vi "HFRR ADV v08.vi"() -> ()   [LabVIEW 2025] (continued)
            n1801 = String To Path(string=w2038) -> (path=w2046:path)
            n1802 = case shown="True" w2037 {
              tunnel: [w2053 w2054] -> w2041
              frame False {
                n1803 = local read "string1"() -> (w2053:string)
              }
              frame True {
                n1804 = local read "String Indicator 4"() -> (w2054:string)
              }
            }
            n1805 = Open/Create/Replace File "Open File"(file path (use dialog)=w2048) -> (refnum out=w2044:refnum<file>)  [unwired: 5 in, 2 out]
            n1806 = Open/Create/Replace File "Open File"(file path (use dialog)=w2047) -> (refnum out=w2043:refnum<file>)  [unwired: 5 in, 2 out]
            n1807 = Open/Create/Replace File "Open File"(file path (use dialog)=w2046) -> (refnum out=w2042:refnum<file>)  [unwired: 5 in, 2 out]
            n1808 = while {
              tunnel: w2044 -> [w2066]
              i -> [w2062]
              stop <- w2061 continue-if-true
              (unwired) TRUE ("line mode (F)")
              n1809 = Read from Text File "Read File"(file (use dialog)=w2066) -> (text=w2063:string)  [unwired: 3 in, 3 out]
              n1810 = local write "Numeric 11"(w2062) -> ()
              n1811 = String Length(string=w2063) -> (length=w2065:i32)
              n1812 = Greater?(x=w2065, y=1) -> (0:w2061:bool)
            }
            n1813 = while {
              tunnel: w2043 -> [w2072]
              i -> [w2068]
              stop <- w2067 continue-if-true
              (unwired) TRUE ("line mode (F)")
              n1814 = Read from Text File "Read File"(file (use dialog)=w2072) -> (text=w2069:string)  [unwired: 3 in, 3 out]
              n1815 = local write "Numeric 12"(w2068) -> ()
              n1816 = String Length(string=w2069) -> (length=w2071:i32)
              n1817 = Greater?(x=w2071, y=1) -> (0:w2067:bool)
            }
            n1818 = while {
              tunnel: w2042 -> [w2078]
              i -> [w2074]
              stop <- w2073 continue-if-true
              (unwired) TRUE ("line mode (F)")
              n1819 = Read from Text File "Read File"(file (use dialog)=w2078) -> (text=w2075:string)  [unwired: 3 in, 3 out]
              n1820 = local write "Numeric 13"(w2074) -> ()
              n1821 = String Length(string=w2075) -> (length=w2077:i32)
              n1822 = Greater?(x=w2077, y=1) -> (0:w2073:bool)
            }
            n1823 = String To Path(string=w2041) -> (path=w2049:path)
            n1824 = Open/Create/Replace File "Open File"(file path (use dialog)=w2049) -> (refnum out=w2045:refnum<file>)  [unwired: 5 in, 2 out]
            n1825 = while {
              tunnel: w2045 -> [w2060]
              i -> [w2056]
              stop <- w2055 continue-if-true
              (unwired) TRUE ("line mode (F)")
              n1826 = Read from Text File "Read File"(file (use dialog)=w2060) -> (text=w2057:string)  [unwired: 3 in, 3 out]
              n1827 = local write "Numeric 8"(w2056) -> ()
              n1828 = String Length(string=w2057) -> (length=w2059:i32)
              n1829 = Greater?(x=w2059, y=1) -> (0:w2055:bool)
            }
          }
          frame #1 {
            w2230 = FALSE ("ACTUAL   MERGE")
            # "Sample Temp"
            # "ECR"
            # "COF"
            # "Time\nCOF\nFF\nTemp"
            n1830 = case shown="True" w2103 {
              tunnel: [w2250 w2251] -> w2104
              frame False {
                n1831 = local read "string1"() -> (w2250:string)
              }
              frame True {
                n1832 = local read "String Indicator 4"() -> (w2251:string)
              }
            }
            n1833 = local read "string1 3"() -> (w2148:string)
            n1834 = String To Path(string=w2104) -> (path=w2235:path)
            n1835 = String To Path(string=w2148) -> (path=w2246:path)
            n1836 = local read "Numeric 12"() -> (w2232:i32)
            n1837 = local read "Numeric 8"() -> (w2234:i32)
            n1838 = local read "string1 2"() -> (w2149:string)
            n1839 = local read "string1 4"() -> (w2147:string)
            n1840 = Open/Create/Replace File "Open File"(file path (use dialog)=w2235) -> (refnum out=w2249:refnum<file>, error out=w2248:errorcluster)  [unwired: 5 in, 1 out]
            n1841 = Open/Create/Replace File "Open File"(file path (use dialog)=w2246) -> (refnum out=w2242:refnum<file>, error out=w2243:errorcluster)  [unwired: 5 in, 1 out]
            n1842 = for {
              N: w2234 -> [_]
              tunnel: w2249 -> [w2397]
              tunnel: w2248 -> [w2396]
              tunnel: [w2386] -> w2161 mode=indexing
              tunnel: [w2384] -> w2218 mode=indexing
              tunnel: [w2385] -> w2213 mode=indexing
              tunnel: w2230 -> [_]
              tunnel: [w2378] -> w2215 mode=indexing
              tunnel: [w2374] -> w2184 mode=indexing
              tunnel: [w2370] -> w2159 mode=indexing
              tunnel: [w2366] -> w2140 mode=indexing
              tunnel: [w2361] -> w2100 mode=indexing
              (unwired) TRUE ("line mode (F)")
              # "freq"
              # "Stroke"
              # "Time"
              # "CoF"
              # "Humidity"
              # "Temp"
              # "Air Temp"
              # "ECR"
              n1843 = Read from Text File "Read File"(file (use dialog)=w2397, error in=w2396) -> (text=w2362:string)  [unwired: 2 in, 3 out]
              n1844 = local write "String 6"(w2362) -> ()
              n1845 = String Subset(string=w2362, offset (0)=0, length (rest)=14 ("length (rest)")) -> (substring=w2390:string)
              n1846 = String Subset(string=w2362, offset (0)=35, length (rest)=9 ("length (rest)")) -> (substring=w2387:string)
              n1847 = String Subset(string=w2362, offset (0)=15, length (rest)=9 ("length (rest)")) -> (substring=w2393:string)
              n1848 = Fract/Exp String To Number(string=w2390) -> (number=w2386:dbl)  [unwired: 3 in, 1 out]
              n1849 = Fract/Exp String To Number(string=w2387) -> (number=w2385:dbl)  [unwired: 3 in, 1 out]
              n1850 = Fract/Exp String To Number(string=w2393) -> (number=w2384:dbl)  [unwired: 3 in, 1 out]
              n1851 = String Subset(string=w2362, offset (0)=85, length (rest)=9 ("length (rest)")) -> (substring=w2363:string)
              n1852 = String Subset(string=w2362, offset (0)=25, length (rest)=9 ("length (rest)")) -> (substring=w2369:string)
              n1853 = String Subset(string=w2362, offset (0)=55, length (rest)=9 ("length (rest)")) -> (substring=w2371:string)
              n1854 = String Subset(string=w2362, offset (0)=45, length (rest)=9 ("length (rest)")) -> (substring=w2377:string)
              n1855 = String Subset(string=w2362, offset (0)=65, length (rest)=9 ("length (rest)")) -> (substring=w2383:string)
              n1856 = Fract/Exp String To Number(string=w2369) -> (number=w2366:dbl)  [unwired: 3 in, 1 out]
              n1857 = Fract/Exp String To Number(string=w2363) -> (number=w2361:dbl)  [unwired: 3 in, 1 out]
              n1858 = Fract/Exp String To Number(string=w2371) -> (number=w2370:dbl)  [unwired: 3 in, 1 out]
              n1859 = Fract/Exp String To Number(string=w2377) -> (number=w2374:dbl)  [unwired: 3 in, 1 out]
              n1860 = Fract/Exp String To Number(string=w2383) -> (number=w2380:dbl)  [unwired: 3 in, 1 out]
              n1861 = Add(x=w2380, y=0.0) -> (x+y=w2378:dbl)
            }
            n1862 = for {
              N: w2232 -> [_]
              tunnel: w2243 -> [w2323]
              tunnel: w2242 -> [w2322]
              tunnel: [w2312] -> w2201 mode=indexing
              tunnel: [w2310] -> w2199 mode=indexing
              tunnel: [w2311] -> w2195 mode=indexing
              tunnel: w2230 -> [_]
              tunnel: [w2304] -> w2197 mode=indexing
              tunnel: [w2300] -> w2179 mode=indexing
              tunnel: [w2296] -> w2155 mode=indexing
              tunnel: [w2293] -> w2136 mode=indexing
              tunnel: [w2289] -> w2095 mode=indexing
              (unwired) 9 ("length (rest)")
              (unwired) 9 ("length (rest)")
              (unwired) TRUE ("line mode (F)")
              n1863 = Read from Text File "Read File"(file (use dialog)=w2322, error in=w2323) -> (text=w2290:string)  [unwired: 2 in, 3 out]
              n1864 = local write "String 8"(w2290) -> ()
              n1865 = String Subset(string=w2290, offset (0)=85) -> (substring=w2292:string)  [unwired: 1 in]
              n1866 = String Subset(string=w2290, offset (0)=35, length (rest)=9 ("length (rest)")) -> (substring=w2313:string)
              n1867 = String Subset(string=w2290, offset (0)=55, length (rest)=9 ("length (rest)")) -> (substring=w2298:string)
              n1868 = String Subset(string=w2290, offset (0)=25) -> (substring=w2294:string)  [unwired: 1 in]
              n1869 = String Subset(string=w2290, offset (0)=15, length (rest)=9 ("length (rest)")) -> (substring=w2319:string)
              n1870 = String Subset(string=w2290, offset (0)=0, length (rest)=14 ("length (rest)")) -> (substring=w2316:string)
              n1871 = String Subset(string=w2290, offset (0)=45, length (rest)=9 ("length (rest)")) -> (substring=w2303:string)
              n1872 = String Subset(string=w2290, offset (0)=65, length (rest)=9 ("length (rest)")) -> (substring=w2309:string)
              n1873 = Fract/Exp String To Number(string=w2292) -> (number=w2289:dbl)  [unwired: 3 in, 1 out]
              n1874 = Fract/Exp String To Number(string=w2313) -> (number=w2311:dbl)  [unwired: 3 in, 1 out]
              n1875 = Fract/Exp String To Number(string=w2298) -> (number=w2296:dbl)  [unwired: 3 in, 1 out]
              n1876 = Fract/Exp String To Number(string=w2294) -> (number=w2293:dbl)  [unwired: 3 in, 1 out]
              n1877 = Fract/Exp String To Number(string=w2319) -> (number=w2310:dbl)  [unwired: 3 in, 1 out]
              n1878 = Fract/Exp String To Number(string=w2316) -> (number=w2312:dbl)  [unwired: 3 in, 1 out]
              n1879 = Fract/Exp String To Number(string=w2303) -> (number=w2300:dbl)  [unwired: 3 in, 1 out]
              n1880 = Fract/Exp String To Number(string=w2309) -> (number=w2306:dbl)  [unwired: 3 in, 1 out]
              n1881 = Add(x=w2306, y=0.0) -> (x+y=w2304:dbl)
            }
            n1882 = String To Path(string=w2149) -> (path=w2247:path)
            n1883 = String To Path(string=w2147) -> (path=w2241:path)
            n1884 = local read "Numeric 11"() -> (w2231:i32)
            n1885 = local read "Numeric 13"() -> (w2233:i32)
            n1886 = Open/Create/Replace File "Open File"(file path (use dialog)=w2247) -> (refnum out=w2245:refnum<file>, error out=w2244:errorcluster)  [unwired: 5 in, 1 out]
            n1887 = Open/Create/Replace File "Open File"(file path (use dialog)=w2241) -> (refnum out=w2240:refnum<file>, error out=w2239:errorcluster)  [unwired: 5 in, 1 out]
            n1888 = for {
              N: w2231 -> [_]
              tunnel: w2245 -> [w2360]
              tunnel: w2244 -> [w2359]
              tunnel: [w2349] -> w2211 mode=indexing
              tunnel: [w2347] -> w2209 mode=indexing
              tunnel: [w2348] -> w2204 mode=indexing
              tunnel: w2230 -> [_]
              tunnel: [w2341] -> w2206 mode=indexing
              tunnel: [w2337] -> w2182 mode=indexing
              tunnel: [w2333] -> w2157 mode=indexing
              tunnel: [w2329] -> w2138 mode=indexing
              tunnel: [w2324] -> w2096 mode=indexing
              (unwired) TRUE ("line mode (F)")
              n1889 = Read from Text File "Read File"(file (use dialog)=w2360, error in=w2359) -> (text=w2325:string)  [unwired: 2 in, 3 out]
              n1890 = local write "String 7"(w2325) -> ()
              n1891 = String Subset(string=w2325, offset (0)=85, length (rest)=9 ("length (rest)")) -> (substring=w2328:string)
              n1892 = String Subset(string=w2325, offset (0)=35, length (rest)=9 ("length (rest)")) -> (substring=w2350:string)
              n1893 = String Subset(string=w2325, offset (0)=55, length (rest)=9 ("length (rest)")) -> (substring=w2336:string)
              n1894 = String Subset(string=w2325, offset (0)=25, length (rest)=9 ("length (rest)")) -> (substring=w2330:string)
              n1895 = String Subset(string=w2325, offset (0)=45, length (rest)=9 ("length (rest)")) -> (substring=w2338:string)
              n1896 = String Subset(string=w2325, offset (0)=0, length (rest)=14 ("length (rest)")) -> (substring=w2353:string)
              n1897 = String Subset(string=w2325, offset (0)=15, length (rest)=9 ("length (rest)")) -> (substring=w2356:string)
              n1898 = String Subset(string=w2325, offset (0)=65, length (rest)=9 ("length (rest)")) -> (substring=w2342:string)
              n1899 = Fract/Exp String To Number(string=w2328) -> (number=w2324:dbl)  [unwired: 3 in, 1 out]
              n1900 = Fract/Exp String To Number(string=w2350) -> (number=w2348:dbl)  [unwired: 3 in, 1 out]
              n1901 = Fract/Exp String To Number(string=w2336) -> (number=w2333:dbl)  [unwired: 3 in, 1 out]
              n1902 = Fract/Exp String To Number(string=w2330) -> (number=w2329:dbl)  [unwired: 3 in, 1 out]
              n1903 = Fract/Exp String To Number(string=w2338) -> (number=w2337:dbl)  [unwired: 3 in, 1 out]
              n1904 = Fract/Exp String To Number(string=w2353) -> (number=w2349:dbl)  [unwired: 3 in, 1 out]
              n1905 = Fract/Exp String To Number(string=w2356) -> (number=w2347:dbl)  [unwired: 3 in, 1 out]
              n1906 = Fract/Exp String To Number(string=w2342) -> (number=w2345:dbl)  [unwired: 3 in, 1 out]
              n1907 = Add(x=w2345, y=0.0) -> (x+y=w2341:dbl)
            }
            n1908 = for {
              N: w2233 -> [_]
              tunnel: w2240 -> [w2288]
              tunnel: w2239 -> [w2287]
              tunnel: [w2277] -> w2193 mode=indexing
              tunnel: [w2276] -> w2186 mode=indexing
              tunnel: w2230 -> [_]
              tunnel: [w2265] -> w2191 mode=indexing
              tunnel: [w2270] -> w2188 mode=indexing
              tunnel: [w2266] -> w2178 mode=indexing
              tunnel: [w2261] -> w2153 mode=indexing
              tunnel: [w2257] -> w2134 mode=indexing
              tunnel: [w2252] -> w2094 mode=indexing
              (unwired) 1.0 ("x")
              (unwired) TRUE ("line mode (F)")
              n1909 = Read from Text File "Read File"(file (use dialog)=w2288, error in=w2287) -> (text=w2253:string)  [unwired: 2 in, 3 out]
              n1910 = local write "String 12"(w2253) -> ()
              n1911 = String Subset(string=w2253, offset (0)=85, length (rest)=9 ("length (rest)")) -> (substring=w2255:string)
              n1912 = String Subset(string=w2253, offset (0)=35, length (rest)=9 ("length (rest)")) -> (substring=w2278:string)
              n1913 = String Subset(string=w2253, offset (0)=55, length (rest)=9 ("length (rest)")) -> (substring=w2263:string)
              n1914 = String Subset(string=w2253, offset (0)=25, length (rest)=9 ("length (rest)")) -> (substring=w2259:string)
              n1915 = String Subset(string=w2253, offset (0)=45, length (rest)=9 ("length (rest)")) -> (substring=w2268:string)
              n1916 = String Subset(string=w2253, offset (0)=15, length (rest)=9 ("length (rest)")) -> (substring=w2284:string)
              n1917 = String Subset(string=w2253, offset (0)=0, length (rest)=14 ("length (rest)")) -> (substring=w2281:string)
              n1918 = String Subset(string=w2253, offset (0)=65, length (rest)=9 ("length (rest)")) -> (substring=w2271:string)
              n1919 = Fract/Exp String To Number(string=w2255) -> (number=w2252:dbl)  [unwired: 3 in, 1 out]
              n1920 = Fract/Exp String To Number(string=w2278) -> (number=w2276:dbl)  [unwired: 3 in, 1 out]
              n1921 = Fract/Exp String To Number(string=w2263) -> (number=w2261:dbl)  [unwired: 3 in, 1 out]
              n1922 = Fract/Exp String To Number(string=w2259) -> (number=w2257:dbl)  [unwired: 3 in, 1 out]
              n1923 = Fract/Exp String To Number(string=w2268) -> (number=w2266:dbl)  [unwired: 3 in, 1 out]
              n1924 = Fract/Exp String To Number(string=w2284) -> (number=w2265:dbl)  [unwired: 3 in, 1 out]
              n1925 = Fract/Exp String To Number(string=w2281) -> (number=w2277:dbl)  [unwired: 3 in, 1 out]
              n1926 = Fract/Exp String To Number(string=w2271) -> (number=w2274:dbl)  [unwired: 3 in, 1 out]
              n1927 = Add(x=w2274, y=0.0) -> (x+y=w2270:dbl)
            }
            n1928 = Delete From Array(array=w2136, index=0) -> (array with subset deleted=w2109:dbl[])  [unwired: 1 in, 1 out]
            n1929 = Delete From Array(array=w2199, index=0) -> (array with subset deleted=w2172:dbl[])  [unwired: 1 in, 1 out]
            n1930 = Delete From Array(array=w2179, index=0) -> (array with subset deleted=w2167:dbl[])  [unwired: 1 in, 1 out]
            n1931 = Delete From Array(array=w2197, index=0) -> (array with subset deleted=w2198:dbl[])  [unwired: 1 in, 1 out]
            n1932 = call-poly <vilib>:"Mean.vi"("X"=w2109) -> ("mean"=→"КОФ2 4":dbl)  [unwired: 1 out]
            n1933 = call-poly <vilib>:"Mean.vi"("X"=w2172) -> ("mean"=→"КОФ3":dbl)  [unwired: 1 out]
            n1934 = call-poly <vilib>:"Mean.vi"("X"=w2167) -> ("mean"=→"CP3":dbl)  [unwired: 1 out]
            n1935 = Delete From Array(array=w2161, index=0) -> (array with subset deleted=w2088:dbl[])  [unwired: 1 in, 1 out]
            n1936 = Delete From Array(array=w2100, index=0) -> (array with subset deleted=w2087:dbl[])  [unwired: 1 in, 1 out]
            n1937 = Delete From Array(array=w2140, index=0) -> (array with subset deleted=w2111:dbl[])  [unwired: 1 in, 1 out]
            n1938 = Delete From Array(array=w2218, index=0) -> (array with subset deleted=w2173:dbl[])  [unwired: 1 in, 1 out]
            n1939 = Delete From Array(array=w2184, index=0) -> (array with subset deleted=w2169:dbl[])  [unwired: 1 in, 1 out]
            "array w/ subset deleted" <- w2169
            n1940 = Delete From Array(array=w2215, index=0) -> (array with subset deleted=w2216:dbl[])  [unwired: 1 in, 1 out]
            n1941 = call-poly <vilib>:"Mean.vi"("X"=w2111) -> ("mean"=→"КОФ2 2":dbl)  [unwired: 1 out]
            n1942 = call-poly <vilib>:"Mean.vi"("X"=w2173) -> ("mean"=→"КОФ1":dbl)  [unwired: 1 out]
            n1943 = Bundle "Bundle"(w2088, w2087) -> (w2093:cluster{dbl[], dbl[]})  [unwired: 1 in]
            n1944 = Bundle "Bundle"(w2088, w2216) -> (w2080:cluster{dbl[], dbl[]})  [unwired: 1 in]
            n1945 = Delete From Array(array=w2095, index=0) -> (array with subset deleted=w2083:dbl[])  [unwired: 1 in, 1 out]
            n1946 = Delete From Array(array=w2096, index=0) -> (array with subset deleted=w2085:dbl[])  [unwired: 1 in, 1 out]
            n1947 = Delete From Array(array=w2206, index=0) -> (array with subset deleted=w2207:dbl[])  [unwired: 1 in, 1 out]
            n1948 = Delete From Array(array=w2094, index=0) -> (array with subset deleted=w2081:dbl[])  [unwired: 1 in, 1 out]
            n1949 = Delete From Array(array=w2188, index=0) -> (array with subset deleted=w2189:dbl[])  [unwired: 1 in, 1 out]
            n1950 = Delete From Array(array=w2213, index=0) -> (array with subset deleted=w2119:dbl[])  [unwired: 1 in, 1 out]
            n1951 = Delete From Array(array=w2159, index=0) -> (array with subset deleted=w2115:dbl[])  [unwired: 1 in, 1 out]
            n1952 = Delete From Array(array=w2195, index=0) -> (array with subset deleted=w2117:dbl[])  [unwired: 1 in, 1 out]
            n1953 = Delete From Array(array=w2155, index=0) -> (array with subset deleted=w2113:dbl[])  [unwired: 1 in, 1 out]
            n1954 = Delete From Array(array=w2204, index=0) -> (array with subset deleted=w2118:dbl[])  [unwired: 1 in, 1 out]
            n1955 = Delete From Array(array=w2157, index=0) -> (array with subset deleted=w2114:dbl[])  [unwired: 1 in, 1 out]
            n1956 = Delete From Array(array=w2138, index=0) -> (array with subset deleted=w2110:dbl[])  [unwired: 1 in, 1 out]
            n1957 = Delete From Array(array=w2182, index=0) -> (array with subset deleted=w2168:dbl[])  [unwired: 1 in, 1 out]
            n1958 = Delete From Array(array=w2209, index=0) -> (array with subset deleted=w2170:dbl[])  [unwired: 1 in, 1 out]
            n1959 = Delete From Array(array=w2186, index=0) -> (array with subset deleted=w2116:dbl[])  [unwired: 1 in, 1 out]
            n1960 = Delete From Array(array=w2153, index=0) -> (array with subset deleted=w2112:dbl[])  [unwired: 1 in, 1 out]
            n1961 = Delete From Array(array=w2134, index=0) -> (array with subset deleted=w2108:dbl[])  [unwired: 1 in, 1 out]
            n1962 = Delete From Array(array=w2178, index=0) -> (array with subset deleted=w2166:dbl[])  [unwired: 1 in, 1 out]
            n1963 = Delete From Array(array=w2191, index=0) -> (array with subset deleted=w2171:dbl[])  [unwired: 1 in, 1 out]
            n1964 = Delete From Array(array=w2201, index=0) -> (array with subset deleted=w2084:dbl[])  [unwired: 1 in, 1 out]
            n1965 = Delete From Array(array=w2211, index=0) -> (array with subset deleted=w2086:dbl[])  [unwired: 1 in, 1 out]
            n1966 = Delete From Array(array=w2193, index=0) -> (array with subset deleted=w2082:dbl[])  [unwired: 1 in, 1 out]
            n1967 = Bundle "Bundle"(w2088, w2119) -> (w2106:cluster{dbl[], dbl[]})  [unwired: 1 in]
            n1968 = Bundle "Bundle"(w2088, w2173) -> (w2107:cluster{dbl[], dbl[]})  [unwired: 1 in]
            n1969 = Bundle "Bundle"(w2119, w2115) -> (w2121:cluster{dbl[], dbl[]})  [unwired: 1 in]
            n1970 = Bundle "Bundle"(w2084, w2083) -> (w2091:cluster{dbl[], dbl[]})  [unwired: 1 in]
            n1971 = Bundle "Bundle"(w2117, w2113) -> (w2123:cluster{dbl[], dbl[]})  [unwired: 1 in]
            n1972 = Bundle "Bundle"(w2084, w2117) -> (w2227:cluster{dbl[], dbl[]})  [unwired: 1 in]
            n1973 = Bundle "Bundle"(w2084, w2113) -> (w2151:cluster{dbl[], dbl[]})  [unwired: 1 in]
            n1974 = Bundle "Bundle"(w2084, w2172) -> (w2237:cluster{dbl[], dbl[]})  [unwired: 1 in]
            n1975 = Bundle "Bundle"(w2084, w2167) -> (w2175:cluster{dbl[], dbl[]})  [unwired: 1 in]
            n1976 = Bundle "Bundle"(w2084, w2198) -> (w2222:cluster{dbl[], dbl[]})  [unwired: 1 in]
            n1977 = Bundle "Bundle"(w2118, w2114) -> (w2122:cluster{dbl[], dbl[]})  [unwired: 1 in]
            n1978 = Bundle "Bundle"(w2086, w2085) -> (w2092:cluster{dbl[], dbl[]})  [unwired: 1 in]
            n1979 = Bundle "Bundle"(w2086, w2118) -> (w2229:cluster{dbl[], dbl[]})  [unwired: 1 in]
            n1980 = Bundle "Bundle"(w2086, w2114) -> (w2152:cluster{dbl[], dbl[]})  [unwired: 1 in]
            n1981 = Bundle "Bundle"(w2086, w2168) -> (w2176:cluster{dbl[], dbl[]})  [unwired: 1 in]
            n1982 = Bundle "Bundle"(w2086, w2170) -> (w2238:cluster{dbl[], dbl[]})  [unwired: 1 in]
            n1983 = Bundle "Bundle"(w2086, w2207) -> (w2220:cluster{dbl[], dbl[]})  [unwired: 1 in]
            n1984 = Bundle "Bundle"(w2116, w2112) -> (w2124:cluster{dbl[], dbl[]})  [unwired: 1 in]
            n1985 = Bundle "Bundle"(w2082, w2081) -> (w2090:cluster{dbl[], dbl[]})  [unwired: 1 in]
            n1986 = Bundle "Bundle"(w2082, w2116) -> (w2228:cluster{dbl[], dbl[]})  [unwired: 1 in]
            n1987 = Bundle "Bundle"(w2082, w2112) -> (w2150:cluster{dbl[], dbl[]})  [unwired: 1 in]
            n1988 = Bundle "Bundle"(w2082, w2166) -> (w2174:cluster{dbl[], dbl[]})  [unwired: 1 in]
            n1989 = Bundle "Bundle"(w2082, w2171) -> (w2236:cluster{dbl[], dbl[]})  [unwired: 1 in]
            n1990 = Bundle "Bundle"(w2082, w2189) -> (w2221:cluster{dbl[], dbl[]})  [unwired: 1 in]
            n1991 = call-poly <vilib>:"Mean.vi"("X"=w2169) -> ("mean"=→"CP1":dbl)  [unwired: 1 out]
            n1992 = call-poly <vilib>:"Mean.vi"("X"=w2110) -> ("mean"=→"КОФ2 3":dbl)  [unwired: 1 out]
            n1993 = call-poly <vilib>:"Mean.vi"("X"=w2168) -> ("mean"=→"CP2":dbl)  [unwired: 1 out]
            n1994 = call-poly <vilib>:"Mean.vi"("X"=w2170) -> ("mean"=→"КОФ2":dbl)  [unwired: 1 out]
            n1995 = call-poly <vilib>:"Mean.vi"("X"=w2108) -> ("mean"=→"КОФ2 5":dbl)  [unwired: 1 out]
            n1996 = call-poly <vilib>:"Mean.vi"("X"=w2166) -> ("mean"=→"CP4":dbl)  [unwired: 1 out]
            n1997 = call-poly <vilib>:"Mean.vi"("X"=w2171) -> ("mean"=→"КОФ4":dbl)  [unwired: 1 out]
            n1998 = Bundle "Bundle"(w2088, w2115) -> (w2079:cluster{dbl[], dbl[]})  [unwired: 1 in]
            n1999 = Bundle "Bundle"(w2088, w2169) -> (w2102:cluster{dbl[], dbl[]})  [unwired: 1 in]
            n2000 = Build Array "Build Array"(w2079, w2102) -> (w2105:cluster{dbl[], dbl[]}[])
            "XY Graph 17" <- w2105
            n2001 = Build Array "Build Array"(w2093, w2092, w2091, w2090) -> (→"Frequency ( Hz )":cluster{dbl[], dbl[]}[])
            n2002 = Build Array "Build Array"(w2121, w2122, w2123, w2124) -> (→"Air Temp ( °C ) vs Humidity ( % RH )":cluster{dbl[], dbl[]}[])
            n2003 = Build Array "Build Array"(w2106, w2229, w2227, w2228) -> (→"Air Temperature  ( °C )":cluster{dbl[], dbl[]}[])
            n2004 = Build Array "Build Array"(w2079, w2152, w2151, w2150) -> (→"Humidity ( %RH )":cluster{dbl[], dbl[]}[])
            n2005 = Build Array "Build Array"(w2107, w2238, w2237, w2236) -> (→"Coefficient Of Friction":cluster{dbl[], dbl[]}[])
            n2006 = Build Array "Build Array"(w2102, w2176, w2175, w2174) -> (→"Sample Temperature ( °C )":cluster{dbl[], dbl[]}[])
            n2007 = Build Array "Build Array"(w2080, w2220, w2222, w2221) -> (→"XY Graph 13":cluster{dbl[], dbl[]}[])
            n2008 = Bundle "Bundle"(w2088, w2111) -> (w2133:cluster{dbl[], dbl[]})  [unwired: 1 in]
            n2009 = Bundle "Bundle"(w2084, w2109) -> (w2131:cluster{dbl[], dbl[]})  [unwired: 1 in]
            n2010 = Bundle "Bundle"(w2086, w2110) -> (w2132:cluster{dbl[], dbl[]})  [unwired: 1 in]
            n2011 = Bundle "Bundle"(w2082, w2108) -> (w2130:cluster{dbl[], dbl[]})  [unwired: 1 in]
            n2012 = Build Array "Build Array"(w2133, w2132, w2131, w2130) -> (→"Stroke ( mm )":cluster{dbl[], dbl[]}[])
            n2013 = local write "XY Graph 16"(w2105) -> ()
          }
          frame #2 {
          }
          frame #3 {
            n2014 = local write "Numeric 8"(0 ("Numeric 8")) -> ()
            n2015 = local write "Numeric 11"(0 ("Numeric 11")) -> ()
            n2016 = local write "Numeric 12"(0 ("Numeric 12")) -> ()
            n2017 = local write "Numeric 13"(0 ("Numeric 13")) -> ()
            n2018 = property on="OPEN" class="Bool (strict)"("Visible"=TRUE) -> ()  [unwired: 2 in, 2 out]
            n2019 = local read "String Control 2"() -> (w2405:string)
            n2020 = local read "String Control 4"() -> (w2404:string)
            n2021 = local read "String Control 6"() -> (w2403:string)
            n2022 = local read "String Control 8"() -> (w2402:string)
            n2023 = Match Pattern(string=w2405, regular expression="Samples / cycle :- ") -> (after substring=w2419:string)  [unwired: 1 in, 3 out]
            n2024 = Match Pattern(string=w2405, regular expression="Frequency :- ") -> (after substring=w2438:string)  [unwired: 1 in, 3 out]
            n2025 = Match Pattern(string=w2404, regular expression="Samples / cycle :- ") -> (after substring=w2415:string)  [unwired: 1 in, 3 out]
            n2026 = Match Pattern(string=w2404, regular expression="Frequency :- ") -> (after substring=w2433:string)  [unwired: 1 in, 3 out]
            n2027 = Match Pattern(string=w2403, regular expression="Samples / cycle :- ") -> (after substring=w2411:string)  [unwired: 1 in, 3 out]
            n2028 = Match Pattern(string=w2403, regular expression="Frequency :- ") -> (after substring=w2428:string)  [unwired: 1 in, 3 out]
            n2029 = Match Pattern(string=w2402, regular expression="Samples / cycle :- ") -> (after substring=w2407:string)  [unwired: 1 in, 3 out]
            n2030 = Match Pattern(string=w2402, regular expression="Frequency :- ") -> (after substring=w2423:string)  [unwired: 1 in, 3 out]
            n2031 = String Subset(string=w2419, length (rest)=6 ("length (rest)")) -> (substring=w2421:string)  [unwired: 1 in]
            n2032 = String Subset(string=w2438, length (rest)=9 ("length (rest)")) -> (substring=w2440:string)  [unwired: 1 in]
            n2033 = String Subset(string=w2415, length (rest)=6 ("length (rest)")) -> (substring=w2417:string)  [unwired: 1 in]
            n2034 = String Subset(string=w2433, length (rest)=9 ("length (rest)")) -> (substring=w2435:string)  [unwired: 1 in]
            n2035 = String Subset(string=w2411, length (rest)=6 ("length (rest)")) -> (substring=w2413:string)  [unwired: 1 in]
            n2036 = String Subset(string=w2428, length (rest)=9 ("length (rest)")) -> (substring=w2430:string)  [unwired: 1 in]
            n2037 = String Subset(string=w2407, length (rest)=6 ("length (rest)")) -> (substring=w2409:string)  [unwired: 1 in]
            n2038 = String Subset(string=w2423, length (rest)=9 ("length (rest)")) -> (substring=w2425:string)  [unwired: 1 in]
            n2039 = Fract/Exp String To Number(string=w2421) -> (number=w2401:dbl)  [unwired: 3 in, 1 out]
            n2040 = Fract/Exp String To Number(string=w2440) -> (number=w2441:dbl)  [unwired: 3 in, 1 out]
            n2041 = Fract/Exp String To Number(string=w2417) -> (number=w2400:dbl)  [unwired: 3 in, 1 out]
            n2042 = Fract/Exp String To Number(string=w2435) -> (number=w2436:dbl)  [unwired: 3 in, 1 out]
            n2043 = Fract/Exp String To Number(string=w2413) -> (number=w2399:dbl)  [unwired: 3 in, 1 out]
            n2044 = Fract/Exp String To Number(string=w2430) -> (number=w2431:dbl)  [unwired: 3 in, 1 out]
            n2045 = Fract/Exp String To Number(string=w2409) -> (number=w2398:dbl)  [unwired: 3 in, 1 out]
            n2046 = Fract/Exp String To Number(string=w2425) -> (number=w2426:dbl)  [unwired: 3 in, 1 out]
            n2047 = local write "sample1"(w2401) -> ()
            n2048 = local write "freq1"(w2441) -> ()
            n2049 = local write "sample2"(w2400) -> ()
            n2050 = local write "freq2"(w2436) -> ()
            n2051 = local write "sample3"(w2399) -> ()
            n2052 = local write "freq3"(w2431) -> ()
            n2053 = local write "sample4"(w2398) -> ()
            n2054 = local write "freq 4"(w2426) -> ()
          }
        }
      }
    }
    n2055 = case shown="True" w1889 {
      selector: w1889 -> [_ w2018]
      frame False {
      }
      frame True {
        n2056 = Not(x=w2018) -> (.not. x?=w2014:bool)
        n2057 = local write "service 3"(w2014) -> ()
        n2058 = local write "OPEN 6"(w2014) -> ()
        n2059 = call <vilib>:"System Exec.vi"("wait until completion? (T)"=TRUE, "command line"="C:\\LAB-IQ\\Scar View.exe") -> ("error out"=→"error out 5":errorcluster)  [unwired: 6 in, 3 out]
      }
    }
    n2060 = case shown="\"Acquire\", Default" w1901 {
      frame "Acquire", Default {
        w2920 = 0.2 ("y")
        w2925 = 1.0 ("y")
        w2926 = 0.8 ("y")
        # "Elapsed time\ncof\nstroke\nAir temp\nTemp\nHumidity"
        n2061 = disable-structure shown="Disabled" {
          frame Disabled {
            n2062 = local read "Flag"() -> (w2943:dbl)
            n2063 = local read "RUN"() -> (w2940:bool)
            n2064 = Not(x=w2940) -> (.not. x?=w2939:bool)
            n2065 = Equal?(x=w2943, y=10.0) -> (x = y?=w2941:bool)
            n2066 = And(x=w2941, y=w2939) -> (x .and. y?=w2938:bool)
            n2067 = case shown="True" w2938 {
              frame False {
              }
              frame True {
                w2944 = FALSE ("Heater Button")
                n2068 = local write "Humidity"(w2944) -> ()
                n2069 = local write "Heater Button"(w2944) -> ()
              }
            }
          }
          frame Enabled {
          }
        }
        n2070 = disable-structure shown="Disabled" {
          frame Disabled {
            n2071 = case shown="True" {
              selector: _ -> [_ _]
              frame False {
              }
              frame True {
                w3035 = TRUE ("Heater")
                n2072 = local write "Humidity"(w3035) -> ()
                n2073 = local write "Heater Button"(w3035) -> ()
                n2074 = local read "TEST STANDARD"() -> (w3038:T4)
                n2075 = local read "TEST STANDARD"() -> (w3033:T4)
                n2076 = Equal?(x=w3038, y=enum16{"ASTM D6079", "ISO 12156", "Custom"}."ISO 12156" ("Test Standard")) -> (x = y?=w3036:bool)
                n2077 = Equal?(x=w3033, y=enum16{"ASTM D6079", "ISO 12156", "Custom"}."ASTM D6079" ("Test Standard")) -> (x = y?=w3032:bool)
                n2078 = case shown="True" w3036 {
                  frame False {
                  }
                  frame True {
                    n2079 = local write "Heater"(TRUE ("Heater")) -> ()
                    n2080 = local write "airtempflg"(FALSE ("airtempflg")) -> ()
                  }
                }
                n2081 = case shown="True" w3032 {
                  frame False {
                  }
                  frame True {
                    n2082 = local write "Heater"(FALSE ("Heater")) -> ()
                    n2083 = local write "airtempflg"(TRUE ("airtempflg")) -> ()
                  }
                }
              }
            }
          }
          frame Enabled {
          }
        }
        n2084 = stacked-sequence {
          frame #0 {
            n2085 = case shown="True" "RST FF" {
              frame False {
              }
              frame True {
                w3101 = 0.0 ("X Scale.Range:Maximum")
                n2086 = property on="Frictional Force ( N )" class="WFChart (strict)"("XScale.Maximum"=600.0 ("X Scale.Range:Maximum"), "XScale.Minimum"=w3101, "YScale.Maximum"=10.0 ("Y Scale.Range:Maximum"), "YScale.Minimum"=w3101) -> ()  [unwired: 2 in, 2 out]
              }
            }
          }
          frame #1 {
            n2087 = case shown="True" "RST TEMP" {
              frame False {
              }
              frame True {
                n2088 = property on="Temperature ( Deg C )" class="WFChart (strict)"("XScale.Minimum"=0.0 ("X Scale.Range:Minimum"), "XScale.Maximum"=600.0 ("X Scale.Range:Maximum"), "YScale.Minimum"=0.0 ("Y Scale.Range:Minimum"), "YScale.Maximum"=100.0 ("Y Scale.Range:Maximum")) -> ()  [unwired: 2 in, 2 out]
              }
            }
          }
          frame #2 {
            n2089 = case shown="True" "RSTCOF" {
              frame False {
              }
              frame True {
                n2090 = property on="Coefficient of Friction" class="WFChart (strict)"("XScale.Minimum"=0.0 ("X Scale.Range:Minimum"), "XScale.Maximum"=600.0 ("X Scale.Range:Maximum"), "YScale.Maximum"=1.0 ("X Scale.Range:Minimum"), "YScale.Minimum"=0.0 ("X Scale.Range:Minimum")) -> ()  [unwired: 2 in, 2 out]
              }
            }
          }
          frame #3 {
            n2091 = case shown="True" "RSTCOF 2" {
              frame False {
              }
              frame True {
                (unwired) 100.0 ("Y Scale.Range:Maximum")
                (unwired) 0.0 ("Y Scale.Range:Minimum")
                (unwired) 600.0 ("X Scale.Range:Maximum")
                (unwired) 0.0 ("X Scale.Range:Minimum")
              }
            }
          }
          frame #4 {
            n2092 = case shown="True" "RSTCOF 3" {
              frame False {
              }
              frame True {
                n2093 = property on="Electrical Contact Resistance ( % )" class="WFChart (strict)"("XScale.Minimum"=0.0 ("X Scale.Range:Minimum"), "XScale.Maximum"=600.0 ("X Scale.Range:Maximum"), "YScale.Minimum"=0.0 ("Y Scale.Range:Minimum"), "YScale.Maximum"=100.0 ("Y Scale.Range:Maximum")) -> ()  [unwired: 2 in, 2 out]
              }
            }
          }
        }
        n2094 = disable-structure shown="Disabled" {
          frame Disabled {
            n2095 = case shown="True" {
              selector: _ -> [_ _]
              frame False {
              }
              frame True {
                n2096 = local read "zflag 2"() -> (w3002:dbl)
                n2097 = local read "yflag"() -> (w3004:dbl)
                n2098 = Equal?(x=w3004, y=2.0 ("tflag")) -> (x = y?=w3006:bool)
                n2099 = Equal?(x=w3002, y=3.0 ("tflag")) -> (x = y?=w3005:bool)
                n2100 = And(x=w3006, y=w3005) -> (x .and. y?=w3000:bool)
                n2101 = case shown="True" w3000 {
                  frame False {
                  }
                  frame True {
                    w3031 = 0.0 ("zflag")
                    n2102 = local write "zflag"(w3031) -> ()
                    n2103 = local write "zflag 2"(w3031) -> ()
                    n2104 = Delete(path (use dialog)=path "C:/LAB-IQ-NXT/WO 2449 TT.sig" ("file path (dialog if empty)")) -> (deleted path=w3030:path)  [unwired: 4 in, 2 out]
                    n2105 = Delete(path (use dialog)=path "C:/LAB-IQ-NXT/WO 2449 TRH.sig" ("file path (dialog if empty)")) -> (deleted path=w3025:path)  [unwired: 4 in, 2 out]
                    n2106 = local read "SEN.RUN HRS"() -> (w3017:dbl)
                    n2107 = local read "SENSOR TIME"() -> (w3015:dbl)
                    n2108 = call <vilib>:"compatOverwrite.vi"("overwrite (F)"=TRUE) -> ("overwrite?"=w3007:T22)
                    n2109 = call <vilib>:"compatOverwrite.vi"("overwrite (F)"=TRUE) -> ("overwrite?"=w3011:T22)
                    n2110 = local read "Total No. of Tests"() -> (w3018:dbl)
                    n2111 = Add(x=w3015, y=w3017) -> (x+y=w3016:dbl)
                    "SEN.RUN HRS" <- w3016
                    n2112 = Open/Create/Replace File(file path (use dialog)=w3030, operation (0:open)=w3007) -> (refnum out=w3008:refnum<file>, error out=w3009:errorcluster)  [unwired: 4 in, 1 out]
                    n2113 = Open/Create/Replace File(file path (use dialog)=w3025, operation (0:open)=w3011) -> (refnum out=w3012:refnum<file>, error out=w3013:errorcluster)  [unwired: 4 in, 1 out]
                    n2114 = Deny Access(4:w3009, 6:T20."deny none" ("deny mode (2)"), 7:w3008) -> (3:w3029:refnum<file>)  [unwired: 1 out]
                    n2115 = Deny Access(4:w3013, 6:T20."deny none" ("deny mode (2)"), 7:w3012) -> (3:w3021:refnum<file>)  [unwired: 1 out]
                    n2116 = Number To Decimal String(number=w3018) -> (decimal integer string=w3026:string)  [unwired: 1 in]
                    n2117 = Number To Decimal String(number=w3016) -> (decimal integer string=w3022:string)  [unwired: 1 in]
                    n2118 = Write to Binary File(file (use dialog)=w3029, data=w3026, 5:FALSE ("prepend array or string size? (T)")) -> ()  [unwired: 3 in, 3 out]
                    n2119 = Write to Binary File(file (use dialog)=w3021, data=w3022, 5:FALSE ("prepend array or string size? (T)")) -> ()  [unwired: 3 in, 3 out]
                  }
                }
              }
            }
          }
          frame Enabled {
          }
        }
        n2120 = local read "RUN"() -> (w2929:bool)
        n2121 = local read "run replace"() -> (w2933:bool)
        n2122 = local read "run replace"() -> (w2932:bool)
        n2123 = case shown="True" w2929 {
          frame False {
            n2124 = local write "run replace"(FALSE ("run replace")) -> ()
          }
          frame True {
            "run replace" <- TRUE ("run replace")
          }
        }
        n2125 = local read "RUN"() -> (w2937:bool)
        n2126 = local read "Set Temp"() -> (w2899:dbl)
        n2127 = local read "SetTemp"() -> (w2901:dbl)
        n2128 = case shown="False" w2937 {
          tunnel: [FALSE ("TEST RUNNING") TRUE ("TEST RUNNING")] -> w2936
          frame False {
            w3120 = 0.0 ("Flag")
            n2129 = local write "Elapsed time"(0.0 ("elapsedtime")) -> ()
            n2130 = local write "Time Remaining"(w3120) -> ()
            n2131 = local write "Flag"(w3120) -> ()
            n2132 = local write "Remaining Time"(w3120) -> ()
          }
          frame True {
            n2133 = local write "Flag"(10.0 ("Flag")) -> ()
          }
        }
        n2134 = case shown="False" w2933 {
          frame False {
            n2135 = local read "zflag"() -> (→"zflag 2":dbl)
            n2136 = local write "yflag"(2.0 ("tflag")) -> ()
            n2137 = local write "FLAG 4"(0.0 ("FLAG")) -> ()
          }
          frame True {
            n2138 = local write "yflag"(1.0 ("tflag")) -> ()
            n2139 = local write "zflag"(3.0 ("zflag")) -> ()
          }
        }
        n2140 = local read "acq 2"() -> (w2931:bool)
        n2141 = local read "AIR TEMP"() -> (w2894:dbl)
        n2142 = local read "Amb temp"() -> (w2898:dbl)
        n2143 = case shown="True" "Save & Continue" {
          frame False {
          }
          frame True {
            "acq 2" <- TRUE ("acq 2")
          }
        }
        n2144 = local read "Set Rh"() -> (w2900:dbl)
        n2145 = Add(x=w2901, y=w2926) -> (x+y=w2927:dbl)
        n2146 = Subtract(x=w2901, y=w2926) -> (x-y=w2928:dbl)
        n2147 = Add(x=w2899, y=w2920) -> (x+y=w2921:dbl)
        n2148 = Subtract(x=w2899, y=w2920) -> (x-y=w2922:dbl)
        n2149 = And(x=w2931, y=w2932) -> (x .and. y?=w2930:bool)
        n2150 = Greater Or Equal?(x=w2894, y=15.0) -> (x >= y?=w2895:bool)
        "powstat" <- w2895
        n2151 = local read "Humidity ( %RH )"() -> (w2897:dbl)
        n2152 = case shown="True" "Save & Continue" {
          frame False {
          }
          frame True {
            n2153 = while {
              tunnel: "0123456789abcdefghijklmnopqrstuvwxyzABCDEFGHIJKLMNOPQRSTUVWXYZ" ("string 2") -> [w3091]
              shift-right: [w3089] -> w3084
              shift-left: "" -> [w3088]
              i -> [w3098]
              stop <- w3097 stop-if-true
              n2154 = Random Number (0-1)() -> (number: 0 to 1=w3092:dbl)
              n2155 = Multiply(x=w3092, y=62.0) -> (x*y=w3094:dbl)
              n2156 = Decrement(x="Length") -> (x-1=w3087:i16)
              n2157 = To Word Integer(number=w3094) -> (16bit integer=w3095:i16)
              n2158 = String Subset(string=w3091, offset (0)=w3095, length (rest)=1 ("length (rest)")) -> (substring=w3090:string)
              n2159 = Greater Or Equal?(x=w3098, y=w3087) -> (x >= y?=w3097:bool)
              n2160 = Concatenate Strings(w3090, w3088) -> (w3089:string)
            }
            n2161 = local write "UUID"(w3084) -> ()
          }
        }
        n2162 = In Range and Coerce(upper limit=w2927, x=w2898, lower limit=w2928) -> (In Range?=w2917:bool)  [unwired: 1 out]
        n2163 = Add(x=w2900, y=w2925) -> (x+y=w2924:dbl)
        n2164 = Subtract(x=w2900, y=w2925) -> (x-y=w2923:dbl)
        n2165 = local read "TEMP"() -> (w2896:dbl)
        n2166 = case shown="True" "Save & Continue" {
          frame False {
          }
          frame True {
            n2167 = local read "Operator ID"() -> (w3425:string)
            n2168 = local read "FILE"() -> (w3431:string)
            n2169 = String Length(string=w3431) -> (length=w3429:i32)
            n2170 = String Length(string=w3425) -> (length=w3426:i32)
            n2171 = Greater?(x=w3429, y=0) -> (0:w3428:bool)
            n2172 = Greater?(x=w3426, y=0) -> (0:w3424:bool)
            n2173 = And(x=w3428, y=w3424) -> (x .and. y?=w3423:bool)
            n2174 = case shown="True" w3423 {
              frame False {
                n2175 = stacked-sequence {
                  frame #0 {
                    n2176 = One Button Dialog(message="Please Enter a File Name and Operator ID to save data !", button name ("OK")="Ok") -> ()  [unwired: 1 out]
                  }
                  frame #1 {
                    n2177 = local write "Save & Continue"(FALSE ("OK Button")) -> ()
                  }
                }
                n2178 = local write "Save & Continue"(FALSE ("OK Button")) -> ()
              }
              frame True {
                n2179 = stacked-sequence {
                  frame #0 {
                    n2180 = call <vilib>:"Application Directory.vi"() -> ("Application Directory"=w3439:path)
                    n2181 = Build Path(base path=w3439, name or relative path="data") -> (appended path=w3438:path)
                    n2182 = local read "FILE"() -> (w3441:string)
                    n2183 = List Folder(path=w3438) -> (folder names=w3437:string[])  [unwired: 3 in, 3 out]
                    n2184 = Equal?(x=w3437, y=w3441) -> (x = y?=w3443:bool[])
                    n2185 = call <vilib>:"Trim Whitespace.vi"("string"=w3441) -> ("trimmed string"=w3436:string)  [unwired: 1 in]
                    n2186 = Or Array Elements(Boolean array=w3443) -> (logical OR=w3442:bool)
                    n2187 = case shown="True" w3442 {
                      tunnel: w3436 -> [_ w3445]
                      frame False {
                      }
                      frame True {
                        w3448 = "_(" ("regular expression")
                        n2188 = Match Pattern(string=w3445, regular expression=w3448) -> (match substring=w3447:string, after substring=w3444:string)  [unwired: 1 in, 2 out]
                        n2189 = Equal?(x=w3447, y=w3448) -> (x = y?=w3446:bool)
                        n2190 = case shown="False" w3446 {
                          tunnel: w3445 -> [w3451 w3461]
                          tunnel: w3444 -> [_ w3463]
                          frame False {
                            n2191 = Concatenate Strings(w3451, "_(" ("regular expression"), "1" ("string"), ")" ("regular expression")) -> (w3449:string)
                            n2192 = local write "FILE"(w3449) -> ()
                          }
                          frame True {
                            n2193 = Decimal String To Number(string=w3463) -> (number=w3462:i32)  [unwired: 2 in, 1 out]
                            n2194 = Search/Split String(string=w3461, search string/char (-)="_(" ("regular expression")) -> (substring before match=w3459:string)  [unwired: 1 in, 2 out]
                            n2195 = Increment(x=w3462) -> (x+1=w3457:i32)
                            n2196 = Number To Decimal String(number=w3457) -> (decimal integer string=w3456:string)  [unwired: 1 in]
                            n2197 = Concatenate Strings(w3459, "_(" ("regular expression"), w3456, ")" ("regular expression")) -> (w3454:string)
                            n2198 = local write "FILE"(w3454) -> ()
                          }
                        }
                      }
                    }
                  }
                  frame #1 {
                    w3475 = 0.0
                    w3477 = cluster{"y":dbl, dbl, "y":dbl}[] [] ("History Data")
                    w3478 = FALSE ("Heater Button")
                    (unwired) ")!" ("string")
                    (unwired) ")" ("string")
                    w3476 = dbl[] [] ("History Data")
                    w3482 = "\r"
                    # "C:\\WinDucom\\Data\\"
                    # "C:\\LAB-IQ-NXT\\data"
                    n2199 = local write "Humidity ( %RH )"(w3475) -> ()
                    n2200 = local write "Frequency ( Hz )"(w3475) -> ()
                    n2201 = local write "speedop"(0.0 ("PIDclk 2")) -> ()
                    n2202 = local write "Set Temp 2"(65.0 ("Set Temp 2")) -> ()
                    n2203 = local write "AIR TEMP"(w3475) -> ()
                    n2204 = local write "clk"(0.0 ("clk")) -> ()
                    n2205 = local write "Stroke 4"(w3475) -> ()
                    n2206 = local write "Stroke"(w3475) -> ()
                    n2207 = local write "COF 3"(w3475) -> ()
                    n2208 = local write "COF 2"(w3475) -> ()
                    n2209 = local write "TEMP"(w3475) -> ()
                    n2210 = local write "ecr 3"(w3475) -> ()
                    n2211 = local write "FF 3"(w3475) -> ()
                    n2212 = local write "FF 2"(w3475) -> ()
                    n2213 = property on="Humidity ( %RH )" class="WFChart (strict)"("History Data"=w3476) -> ()  [unwired: 2 in, 2 out]
                    n2214 = property on="Coefficient of Friction" class="WFChart (strict)"("History Data"=w3476) -> ()  [unwired: 2 in, 2 out]
                    n2215 = property on="Coefficient of Friction" class="WFChart (strict)"("History Data"=w3476) -> ()  [unwired: 2 in, 2 out]
                    n2216 = property on="Frictional Force ( N )" class="WFChart (strict)"("History Data"=w3476) -> ()  [unwired: 2 in, 2 out]
                    n2217 = property on="Electrical Contact Resistance ( % )" class="WFChart (strict)"("History Data"=w3476) -> ()  [unwired: 2 in, 2 out]
                    n2218 = property on="Electrical Contact Resistance ( % )" class="WFChart (strict)"("History Data"=w3476) -> ()  [unwired: 2 in, 2 out]
                    n2219 = property on="Temperature ( Deg C )" class="WFChart (strict)"("History Data"=w3476) -> ()  [unwired: 2 in, 2 out]
                    n2220 = property on="Frictional Force ( N )" class="WFChart (strict)"("History Data"=w3476) -> ()  [unwired: 2 in, 2 out]
                    n2221 = property on="Coefficient of Friction" class="WFChart (strict)"("History Data"=w3476) -> ()  [unwired: 2 in, 2 out]
                    n2222 = property on="Frictional Force ( N )" class="WFChart (strict)"("History Data"=w3476) -> ()  [unwired: 2 in, 2 out]
                    n2223 = property on="Electrical Contact Resistance ( % )" class="WFChart (strict)"("History Data"=w3476) -> ()  [unwired: 2 in, 2 out]
                    n2224 = property on="Temperature ( Deg C )" class="WFChart (strict)"("History Data"=w3476) -> ()  [unwired: 2 in, 2 out]
                    n2225 = property on="Humidity ( %RH )" class="WFChart (strict)"("History Data"=w3476) -> ()  [unwired: 2 in, 2 out]
                    n2226 = property on="Stroke ( mm )" class="WFChart (strict)"("History Data"=w3477) -> ()  [unwired: 2 in, 2 out]
                    n2227 = property on="Stroke ( mm )" class="WFChart (strict)"("History Data"=w3477) -> ()  [unwired: 2 in, 2 out]
                    n2228 = local write "Humidity"(w3478) -> ()
                    n2229 = local write "Heater Button"(w3478) -> ()
                    n2230 = local read "FILE"() -> (w3471:string)
                    n2231 = local read "NORMAL LOAD"() -> (w3497:dbl)
                    n2232 = call "file check.vi"("file name in"=w3471) -> ("error out"=w3474:errorcluster, "file name out"=w3468:string)  [unwired: 9 in]
                    n2233 = call "FILE PATH CREATION.vi"("error in"=w3474, "FILE NAME :"=w3468) -> ("FILE OUT"=w3467:path)  [unwired: 8 in, 1 out]
                    n2234 = Concatenate Strings(w3468, ".dgf" ("Substring")) -> (w3473:string)
                    n2235 = Concatenate Strings(w3468, ".duf" ("Substring")) -> (w3469:string)
                    n2236 = Multiply(x=w3497, y=1.0) -> (x*y=w3496:dbl)
                    n2237 = Build Path(base path=w3467, name or relative path=w3473) -> (appended path=w3466:path)
                    n2238 = Build Path(base path=w3467, name or relative path=w3469) -> (appended path=w3465:path)
                    n2239 = Number To Fractional String(number=w3496, width (-)=i16 5, precision (6)=i16 2) -> (F-format string=w3505:string)  [unwired: 1 in]
                    n2240 = local read "Fuel Discription :"() -> (w3492:string)
                    n2241 = local read "Batch Ref Num :"() -> (w3480:string)
                    n2242 = Get Date/Time String(date format (0)=enum16{"short", "long", "abbreviated"}."short") -> (date string=w3516:string, time string=w3513:string)  [unwired: 2 in]
                    n2243 = local read "Remarks :"() -> (w3491:string)
                    n2244 = Concatenate Strings("Load :- " ("Substring"), w3505, " N ," ("Substring")) -> (w3504:string)
                    n2245 = local read "String 41"() -> (w3483:string)
                    n2246 = Concatenate Strings(w3492) -> (w3493:string)
                    n2247 = Concatenate Strings(w3480) -> (w3479:string)
                    n2248 = Concatenate Strings("tested by") -> (w3487:string)
                    n2249 = Concatenate Strings("(" ("Substring"), w3516, ")" ("Substring"), w3513) -> (w3485:string)
                    "concatenated string" <- w3485
                    n2250 = Concatenate Strings(w3491, "," ("string")) -> (w3490:string)
                    n2251 = Concatenate Strings("  TIME;      COF;       STROKE;     AIR TEMP;  TEMP;  HUMIDITY;  ECR; PID-OUT; FREQUENCY" ("Substring"), "\r") -> (w3500:string)
                    n2252 = Concatenate Strings(w3483, w3482, "Fuel Discription :-" ("Substring"), w3493, w3482, w3504, w3482, "Batch Ref Num :-" ("Substring"), w3479, w3482, " Remarks :- " ("Substring"), w3490, w3482, " Date :- " ("Substring"), w3485, w3482, "Tested By :-" ("Substring"), w3487) -> (w3498:string)
                    "REMARKS" <- w3498
                    n2253 = call <vilib>:"Write Characters To File.vi"("append to file? (new file:F)"=FALSE, "character string"=w3500, "file path (dialog if empty)"=w3466) -> ()  [unwired: 2 in, 1 out]
                    n2254 = call <vilib>:"Write Characters To File.vi"("append to file? (new file:F)"=FALSE, "character string"=w3498, "file path (dialog if empty)"=w3465) -> ()  [unwired: 2 in, 1 out]
                  }
                  frame #2 {
                    n2255 = local write "Cycles elapsed"(0 ("Cycles elapsed")) -> ()
                    n2256 = local write "cyclecount"(0 ("cyclecount")) -> ()
                    n2257 = local write "Save & Continue"(FALSE ("OK")) -> ()
                    n2258 = local write "autostrtflg"(TRUE ("autostrtflg")) -> ()
                    n2259 = local write "Save"(FALSE ("Save")) -> ()
                    n2260 = Get Date/Time In Seconds() -> (seconds since 1Jan1904=w3522:timestamp)
                    n2261 = To Double Precision Float(number=w3522) -> (double precision float=w3521:dbl)
                    n2262 = local write "acq timer"(w3521) -> ()
                    n2263 = One Button Dialog(message="Please ensure sample is mounted properly and machine is ready in all aspects for testing !", button name ("OK")="Ok") -> ()  [unwired: 1 out]
                  }
                  frame #3 {
                    n2264 = stacked-sequence {
                      frame #0 {
                        n2265 = local write "Main Dashboard Buttons"(T2."Dashboard" ("Main Dashboard Buttons")) -> ()
                        n2266 = local write "Main Tab"(T3."Acquire" ("Main Tab")) -> ()
                      }
                      frame #1 {
                        n2267 = local write "EVENT LOG"("" ("EVENT LOG")) -> ()
                      }
                      frame #2 {
                        n2268 = Wait (ms)(milliseconds to wait=u32 50) -> ()  [unwired: 1 out]
                      }
                      frame #3 {
                        n2269 = disable-structure shown="Disabled" {
                          frame Disabled {
                            n2270 = local read "EVENT LOG"() -> (w3533:string)
                            n2271 = call "Event Log.vi"("Content"="Test Details", "EVENT LOG"=w3533) -> ("EVENT LOG"=w3532:string)  [unwired: 8 in, 1 out]
                            n2272 = local write "EVENT LOG"(w3532) -> ()
                          }
                          frame Enabled {
                          }
                        }
                      }
                      frame #4 {
                        n2273 = Wait (ms)(milliseconds to wait=u32 50) -> ()  [unwired: 1 out]
                      }
